vi "Launch SubPanel.vi"(7 "Sensor Type":T3, 8 "error in":errorcluster, 9 "Sub Panel":refnum<vi>, 10 "Board Info for checking":T1, 11 "Item Ref in":T2 format="%.0x") -> (0 "error out":errorcluster, 2 "VI Refnum":refnum<vi>, 3 "Item Ref out":T2 format="%.0x")   [LabVIEW 2011, in "PXIe-433x Custom Device.lvlib"]
uses:
  PXIe-433x Custom Device.lvlib
  Sensor Type.ctl
  <vilib>/NI Veristand/Custom Device API/Custom Device Item Ref.ctl
  Board Info for checking settings.ctl
  <vilib>/NI Veristand/Custom Device API/Custom Device API.lvlib
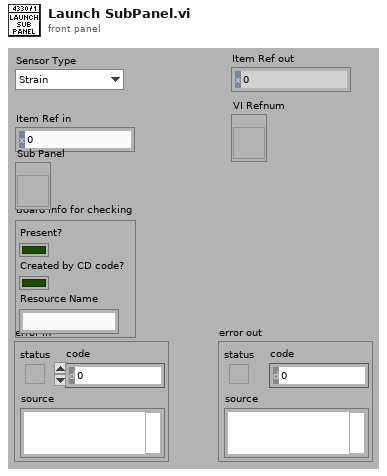
[diagram p1: front panel]
types:
  T1 = typedef "PXIe-433x Custom Device.lvlib/Board Info for checking settings.ctl" = cluster{"Present?":bool, "Created by CD code?":bool, "Resource Name":string}
  T2 = typedef "Custom Device API.lvlib/Custom Device Item Ref.ctl" = u64
  T3 = typedef "PXIe-433x Custom Device.lvlib/Sensor Type.ctl" = enum16{"Strain", "Force", "Pressure", "Torque"}
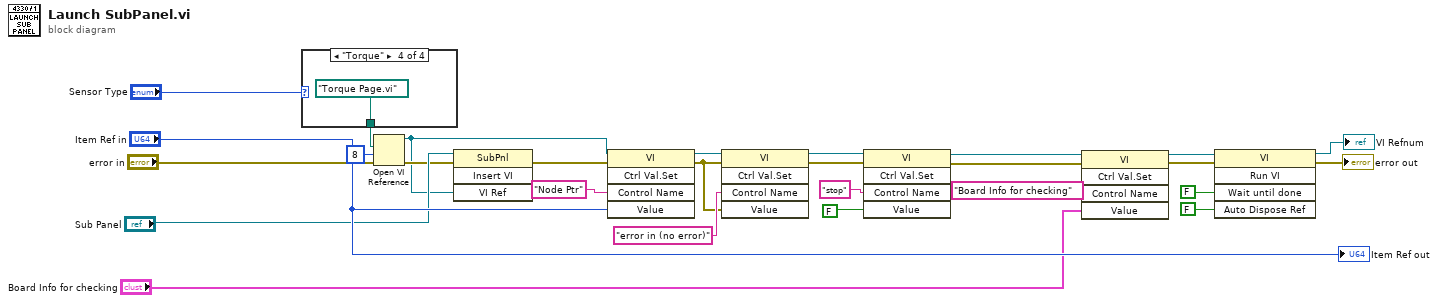
[diagram p0: block diagram]
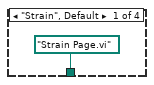
[diagram p2: hidden frame]
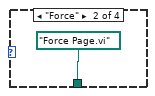
[diagram p3: hidden frame]
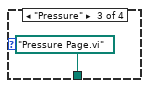
[diagram p4: hidden frame]
diagram:
  n1 = case shown="\"Torque\"" "Sensor Type" {
    tunnel: [path "Strain Page.vi" ("vi path") path "Force Page.vi" ("vi path") path "Pressure Page.vi" ("vi path") path "Torque Page.vi" ("vi path")] -> w1
    frame "Strain", Default {
    }
    frame "Force" {
    }
    frame "Pressure" {
    }
    frame "Torque" {
    }
  }
  n2 = Open VI Reference(vi path=w1, options=8, error in (no error)="error in") -> (vi reference=w3:refnum<vi>, error out=w4:errorcluster)  [unwired: 3 in]
  n3 = invoke on="Invoke Node" class="SubPnl" method="Insert VI"(reference="Sub Panel", error in=w4, "VI Ref"=w3) -> (error out=w6:errorcluster)  [unwired: 1 in, 3 out]
  n4 = invoke class="VI" method="Ctrl Val.Set"(reference=w3, error in=w6, "Control Name"="Node Ptr", "Value"="Item Ref in") -> (reference out=w16:refnum<vi>, error out=w17:errorcluster)  [unwired: 1 in, 3 out]
  n5 = invoke class="VI" method="Ctrl Val.Set"(reference=w16, error in=w17, "Control Name"="error in (no error)", "Value"=w17) -> (reference out=w14:refnum<vi>, error out=w13:errorcluster)  [unwired: 1 in, 3 out]
  n6 = invoke class="VI" method="Ctrl Val.Set"(reference=w14, error in=w13, "Control Name"="stop", "Value"=FALSE ("Wait Until Done")) -> (reference out=w10:refnum<vi>, error out=w9:errorcluster)  [unwired: 1 in, 3 out]
  n7 = invoke class="VI" method="Ctrl Val.Set"(reference=w10, error in=w9, "Control Name"="Board Info for checking", "Value"="Board Info for checking") -> (reference out=w8:refnum<vi>, error out=w5:errorcluster)  [unwired: 1 in, 3 out]
  n8 = invoke class="VI" method="Run VI"(reference=w8, error in=w5, "Wait until done"=FALSE ("Wait Until Done"), "Auto Dispose Ref"=FALSE ("Auto Dispose Reference")) -> (reference out=→"VI Refnum":refnum<vi>, error out=→"error out":errorcluster)  [unwired: 1 in, 3 out]
  "Item Ref out" <- "Item Ref in"
